vi "NF WF1973_74 TRIG Sel.vi"(8 "error in (no error)":errorcluster caption="Error IN", 9 "Mode(Start)":u16(ring) items=["Start", "Stop", "Hold(Sweep & Sequence)", "Resume(Sweep & Sequence)", "Ebranch(Sequence)", "Sbranch(Sequence)", "IStop(Sequence)"], 10 "Ch(Ch1)":bool, 11 "VISAsession":refnum<visa-resource-name>) -> (0 "error out":errorcluster caption="Error OUT", 3 "CopyVISAsession":refnum<visa-resource-name>)   [LabVIEW 2010]
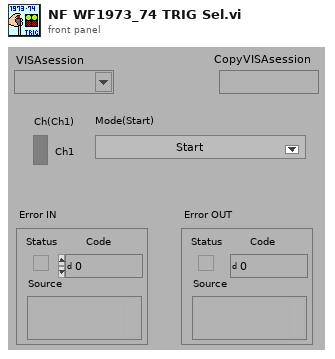
[diagram p1: front panel]
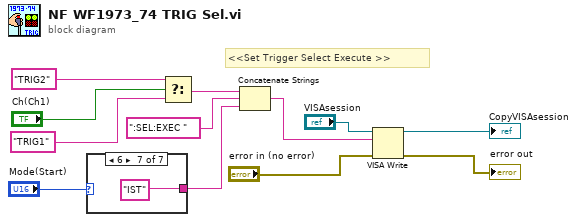
[diagram p0: block diagram]
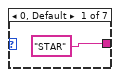
[diagram p2: hidden frame]
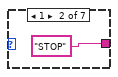
[diagram p3: hidden frame]
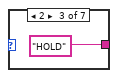
[diagram p4: hidden frame]
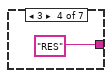
[diagram p5: hidden frame]
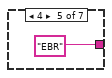
[diagram p6: hidden frame]
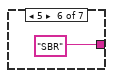
[diagram p7: hidden frame]
diagram:
  # "<<Set Trigger Select Execute >>"
  n1 = case shown="6" "Mode(Start)" {
    tunnel: ["STAR" ("文字列") "STOP" ("文字列") "HOLD" ("文字列") "RES" ("文字列") "EBR" ("文字列") "SBR" ("文字列") "IST" ("文字列")] -> w1
    frame 0, Default {
    }
    frame 1 {
    }
    frame 2 {
    }
    frame 3 {
    }
    frame 4 {
    }
    frame 5 {
    }
    frame 6 {
    }
  }
  n2 = Select(t="TRIG2" ("文字列"), s="Ch(Ch1)", f="TRIG1" ("文字列")) -> (s? t:f=w5:string)
  n3 = Concatenate Strings(w5, ":SEL:EXEC " ("文字列"), w1) -> (w3:string)
  n4 = VISA Write(VISA resource name="VISAsession", write buffer=w3, error in (no error)="error in (no error)") -> (VISA resource name out=→"CopyVISAsession":refnum<visa-resource-name>, error out=→"error out":errorcluster)  [unwired: 1 out]
